vi "user input.vi"(8 "error in":errorcluster, 11 "Interface":T1) -> (0 "error out":errorcluster, 3 "Inputs from system":T3)   [LabVIEW 2017, in "ScaleAndLimitModule runtime.lvclass"]
uses:
  ScaleAndLimitModule runtime.lvclass
  input user data.ctl
  <vilib>/NI/PowerElectronicsControl/ScaleAndLimit/Interface/Interface.ctl
  <instrlib>/_niInstr/Instruction Framework/v1/Host/Instruction Target/niInstr Instruction Target v1 Host.lvclass
  <instrlib>/_niInstr/Instruction Framework/v1/Host/Instruction Framework Context/niInstr Instruction Framework Context v1 Host.lvclass
  <vilib>/NI/PowerElectronicsControl/ScaleAndLimit/Interface/Configuration.ctl
  <vilib>/NI/PowerElectronicsControl/ScaleAndLimit/Interface/ScaleAndLimitInterface.lvlib
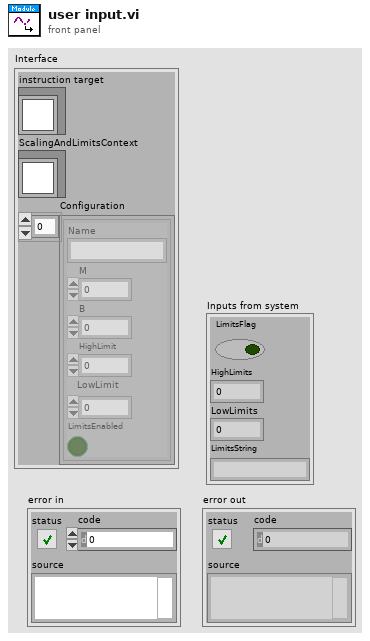
[diagram p1: front panel]
types:
  T1 = typedef "ScaleAndLimitInterface.lvlib/Interface.ctl" = cluster{"instruction target":refnum<class "niInstr Instruction Target v1 Host.lvclass">, "ScalingAndLimitsContext":refnum<class "niInstr Instruction Framework Context v1 Host.lvclass">, "Configuration":T2[]}
  T2 = typedef "ScaleAndLimitInterface.lvlib/Configuration.ctl" = cluster{"Name":string, "M":dbl, "B":i16, "HighLimit":dbl, "LowLimit":dbl, "LimitsEnabled":bool}
  T3 = typedef "ScaleAndLimitModule runtime.lvclass/input user data.ctl" = cluster{"LimitsFlag":bool, "HighLimits":u16, "LowLimits":u16, "LimitsString":string}
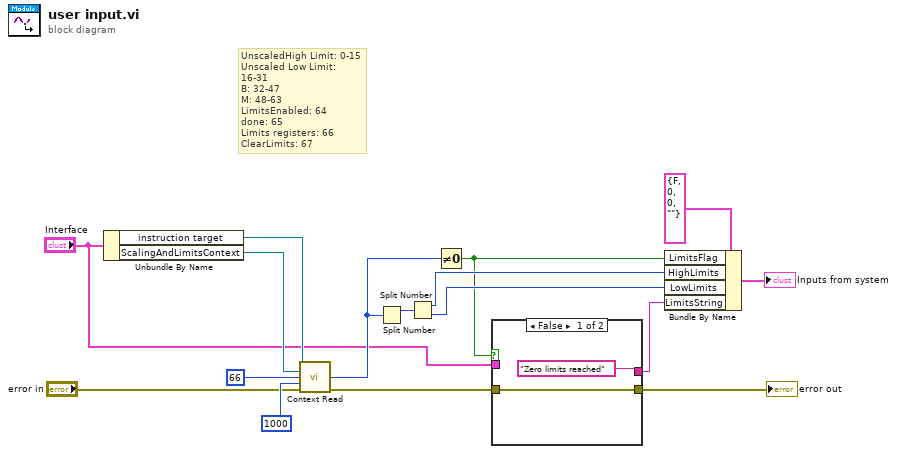
[diagram p0: block diagram]
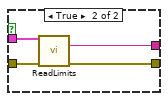
[diagram p2: hidden frame]
diagram:
  # "UnscaledHigh Limit: 0-15\nUnscaled Low Limit: 16-31\nB: 32-47\nM: 48-63\nLimitsEnabled: 64\ndone: 65\nLimits registers: 66\nClearLimits: 67"
  n1 = Unbundle By Name("Interface") -> ("instruction target"=w8:refnum<class "niInstr Instruction Target v1 Host.lvclass">, "ScalingAndLimitsContext"=w7:refnum<class "niInstr Instruction Framework Context v1 Host.lvclass">)
  n2 = call <instrlib>:"Context Read.vi"("instruction target in"=w8, "context in"=w7, "address"=u64 66, "timeout (5000 ms)"=1000, "error in"="error in") -> ("data"=w11:u64, "error out"=w6:errorcluster)  [unwired: 7 in, 2 out]
  n3 = Split Number(x=w11) -> (hi(x)=w12:u32)  [unwired: 1 out]
  n4 = Split Number(x=w12) -> (hi(x)=w10:u16, lo(x)=w9:u16)
  n5 = Not Equal To 0?(x=w11) -> (x != 0?=w4:bool)
  n6 = case shown="False" w4 {
    tunnel: w6 -> [w17 w22]
    tunnel: [w17 w21] -> w5
    tunnel: "Interface" -> [_ w20]
    tunnel: ["Zero limits reached" w19] -> w2
    frame False {
    }
    frame True {
      n7 = call <vilib>:"ReadLimits.vi"("Interface in"=w20, "error in (no error)"=w22) -> ("Limits"=w19:string, "error out"=w21:errorcluster)  [unwired: 11 in, 1 out]
    }
  }
  "error out" <- w5
  n8 = Bundle By Name(cluster=T3 {"LimitsFlag"=FALSE, "HighLimits"=0, "LowLimits"=0, "LimitsString"=""} ("Inputs from system"), "LimitsFlag"=w4, "HighLimits"=w10, "LowLimits"=w9, "LimitsString"=w2) -> (→"Inputs from system":T3)
